vi "decrement counter.vi"   [LabVIEW 2018]
uses:
  State Machine/State Machine.lvclass
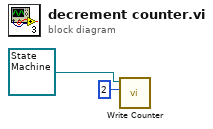
[diagram p0: block diagram]
diagram:
  n1 = call "Write Counter.vi"("Counter"=u16 2, "State Machine in"=refnum<class "State Machine.lvclass"> refnum ("State Machine.lvclass")) -> ()  [unwired: 8 in, 2 out]
